vi "Action.vi"(8 "b":dbl, 10 "a":dbl, 11 "Root in":refnum<class "Root.lvclass">) -> (1 "result":dbl, 3 "Root out":refnum<class "Root.lvclass">)   [LabVIEW 2020, in "Root.lvlib" / "Root.lvclass"]
uses:
  Root.lvclass
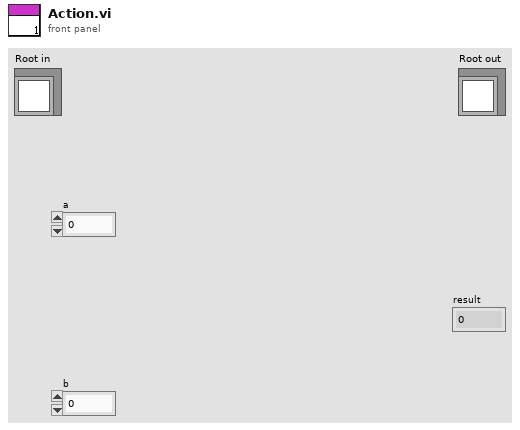
[diagram p1: front panel]
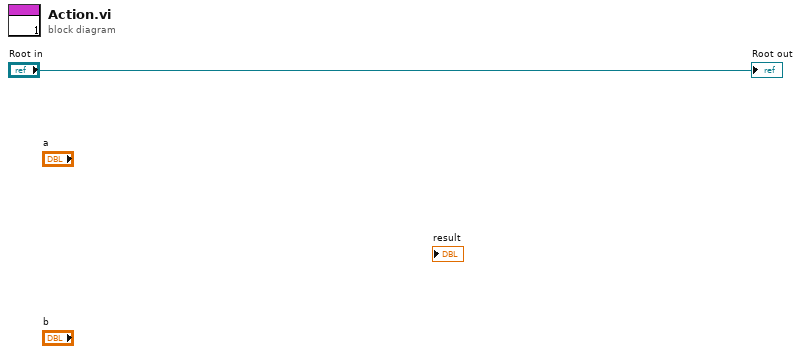
[diagram p0: block diagram]
diagram:
  "Root out" <- "Root in"
